vi "读取串口数据.vi"(8 "error in (no error)":errorcluster caption="错误输入（无错误）", 11 "硬件 输入":refnum<class "硬件.lvclass">) -> (0 "error out":errorcluster caption="错误输出", 2 "读取到的内容":string, 3 "硬件 输出":refnum<class "硬件.lvclass">)   [LabVIEW 2015, in "硬件.lvlib" / "硬件.lvclass"]
uses:
  <vilib>/Instr/_visa.llb/VISA Configure Serial Port (Instr).vi
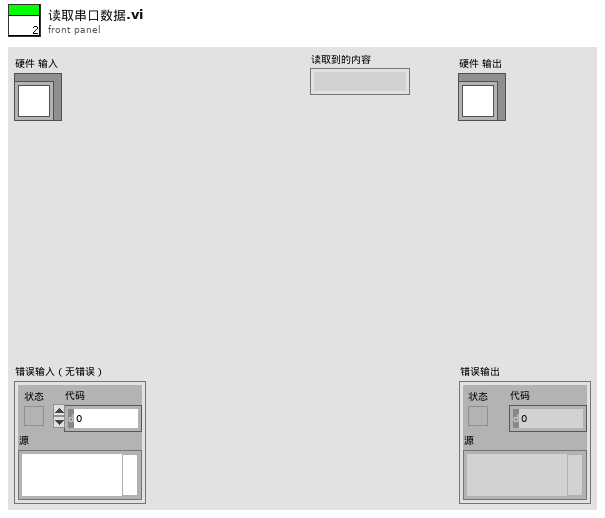
[diagram p1: front panel]
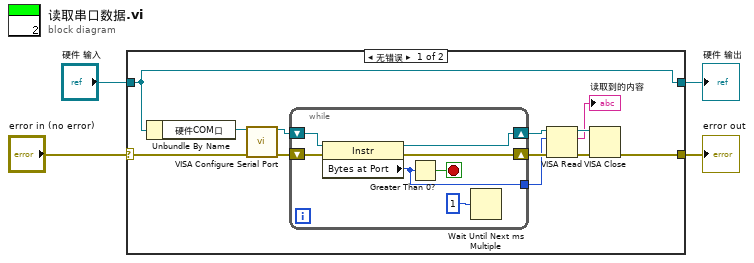
[diagram p0: block diagram]
diagram:
  n1 = case shown="无错误" "error in (no error)" {
    selector: "error in (no error)" -> [w13 w25]
    tunnel: [w12 w25] -> w3
    tunnel: [w16 w24] -> w1
    tunnel: "硬件 输入" -> [w16 w24]
    frame No Error {
      n2 = Unbundle By Name(w16) -> ("硬件COM口"=w15:refnum<visa-resource-name>)
      n3 = call-poly "VISA Configure Serial Port"("VISA resource name"=w15, "error in (no error)"=w13) -> ("VISA resource name out"=w7:refnum<visa-resource-name>, "error out"=w6:errorcluster)  [unwired: 12 in]
      n4 = while {
        tunnel: [w18] -> w8
        shift-right: [w23] -> w10
        shift-left: w7 -> [w21]
        shift-right: [w22] -> w9
        shift-left: w6 -> [w20]
        stop <- w19 stop-if-true
        n5 = property class="Instr"(reference=w21, error in=w20) -> (reference out=w23:refnum<visa-resource-name>, error out=w22:errorcluster, "Bytes at Port"=w18:u32)
        n6 = Greater Than 0?(x=w18) -> (x > 0?=w19:bool)
        n7 = Wait Until Next ms Multiple(millisecond multiple=u32 1 ("毫秒倍数")) -> ()  [unwired: 1 out]
      }
      n8 = VISA Read(VISA resource name=w10, byte count=w8, error in (no error)=w9) -> (VISA resource name out=w14:refnum<visa-resource-name>, read buffer=→"读取到的内容":string, error out=w11:errorcluster)  [unwired: 1 out]
      n9 = VISA Close(VISA resource name=w14, error in (no error)=w11) -> (error out=w12:errorcluster)
    }
    frame Error {
    }
  }
  "error out" <- w3
  "硬件 输出" <- w1
